vi "HV_reopen.vi"(9 "Serial Configuration":T1={"Baud Rate"=9600, "Parity"=0, "Data Bits"=8, "Stop Bits"=10, "Flow Control"=0} {"Flow Control" items=["None", "XON/XOFF", "RTS/CTS", "XON/XOFF & RTS/CTS", "DTR/DSR", "XON/XOFF & DTR/DSR"]; "Stop Bits" items=["1.0"=10, "1.5"=15, "2.0"=20]; "Data Bits" items=["7"=7, "8"=8]; "Parity" items=["None", "Odd", "Even", "Mark", "Space"]; "Baud Rate" items=["300"=300, "600"=600, "1200"=1200, "2400"=2400, "4800"=4800, "9600"=9600, "19200"=19200]}, 11 "VISA resource name":refnum<visa-resource-name>) -> (0 "error out":errorcluster, 3 "VISA resource name out":refnum<visa-resource-name>)   [LabVIEW 2015, in "VIPM2.lvlib"]
uses:
  VIPM2.lvlib
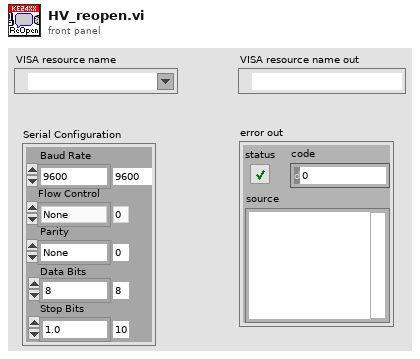
[diagram p1: front panel]
types:
  T1 = cluster{"Baud Rate":u32, "Parity":u16, "Data Bits":u16, "Stop Bits":u16, "Flow Control":u16}
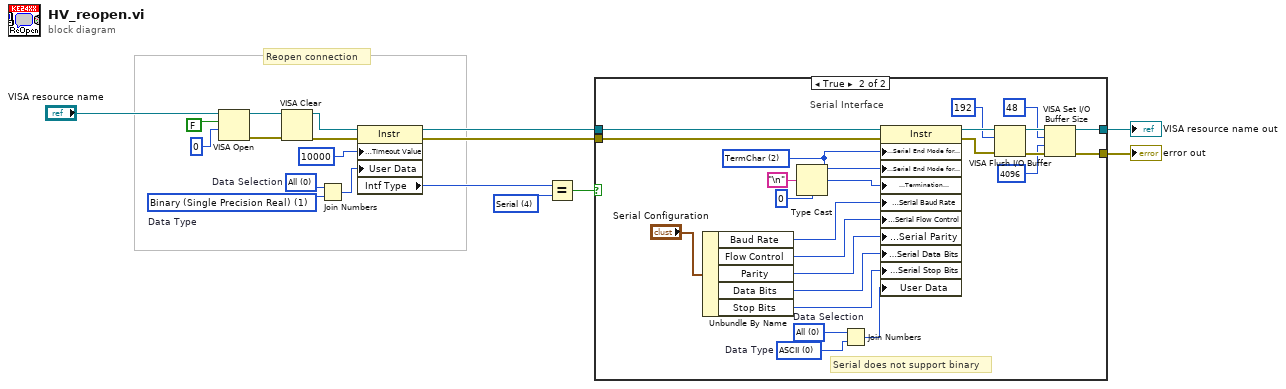
[diagram p0: block diagram]
diagram:
  w3 = u16 4 items=["GPIB"=1, "VXI"=2, "GPIB-VXI"=3, "Serial"=4, "PXI"=5, "TCPIP"=6, "USB"=7] ("Interface Information:Interface Type")
  w11 = u16 1 items=["ASCII", "Binary (Single Precision Real)"]  # Data Type
  w12 = u16 0 items=["All", "Volt and Amp", "Volt", "Amp"]  # Data Selection
  # "Reopen connection"
  n1 = VISA Open(duplicate session (F)=FALSE, access mode=u32 0, VISA resource name="VISA resource name") -> (VISA resource name=w16:refnum<visa-resource-name>, error out=w15:errorcluster)  [unwired: 2 in]
  n2 = VISA Clear(VISA resource name=w16, error in (no error)=w15) -> (VISA resource name out=w14:refnum<visa-resource-name>, error out=w13:errorcluster)
  n3 = Join Numbers(hi=w12, lo=w11) -> ((hi.lo)=w10:u32)
  n4 = property class="Instr"(reference=w14, error in=w13, "General Settings:Timeout Value"=u32 10000, "User Data"=w10) -> (reference out=w6:refnum<visa-resource-name>, error out=w7:errorcluster, "Intf Type"=w2:u16)
  n5 = Equal?(x=w2, y=w3) -> (x = y?=w1:bool)
  n6 = case shown="True" w1 {
    tunnel: [w19 w41] -> w5
    tunnel: [w20 w38] -> w4
    tunnel: w6 -> [w19 w43]
    tunnel: w7 -> [w20 w44]
    frame False {
      # "GPIB"
    }
    frame True {
      w23 = u16 0 items=["ASCII", "Binary (Single Precision Real)"]  # Data Type
      w21 = u16 0 items=["All", "Volt and Amp", "Volt", "Amp"]  # Data Selection
      w31 = u16 2 items=["None", "LastBit", "TermChar"] ("Serial Settings:Serial End Mode for Reads")
      # "Serial does not support binary"
      # "Serial Interface"
      n7 = Unbundle By Name("Serial Configuration") -> ("Baud Rate"=w29:u32, "Flow Control"=w25:u16, "Parity"=w27:u16, "Data Bits"=w28:u16, "Stop Bits"=w24:u16)
      n8 = Type Cast(type=u8 0, x="\n" ("Line Feed Constant")) -> (*(type *) &x=w30:u8)
      n9 = Join Numbers(hi=w21, lo=w23) -> ((hi.lo)=w22:u32)
      n10 = property class="Instr"(reference=w43, error in=w44, "Serial Settings:Serial End Mode for Reads"=w31, "Serial Settings:Serial End Mode for Writes"=w31, "Message Based Settings:Termination Character"=w30, "Serial Settings:Serial Baud Rate"=w29, "Serial Settings:Serial Flow Control"=w25, "Serial Settings:Serial Parity"=w27, "Serial Settings:Serial Data Bits"=w28, "Serial Settings:Serial Stop Bits"=w24, "User Data"=w22) -> (reference out=w37:refnum<visa-resource-name>, error out=w40:errorcluster)
      n11 = VISA Flush I/O Buffer(VISA resource name=w37, mask (16)=u16 192, error in (no error)=w40) -> (VISA resource name out=w42:refnum<visa-resource-name>, error out=w39:errorcluster)
      n12 = VISA Set I/O Buffer Size(VISA resource name=w42, mask (16)=u16 48, size (4096)=u32 4096 ("size (0)"), error in (no error)=w39) -> (VISA resource name out=w41:refnum<visa-resource-name>, error out=w38:errorcluster)
    }
  }
  "VISA resource name out" <- w5
  "error out" <- w4
